vi "name.vi"(0 "Name in":string, 5 "IN VARIANT in":variant) -> (4 "Name":string, 6 "IN VARIANT out":variant)   [LabVIEW 2015]
uses:
  <vilib>/Utility/Data Type/NI_Data Type.lvlib
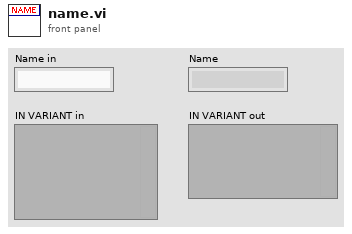
[diagram p1: front panel]
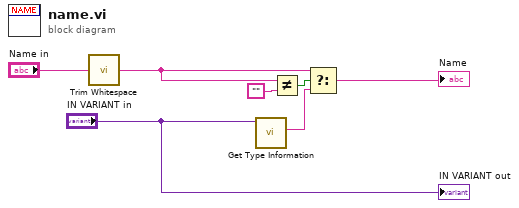
[diagram p0: block diagram]
diagram:
  n1 = call <vilib>:"Trim Whitespace.vi"("string"="Name in") -> ("trimmed string"=w6:string)  [unwired: 1 in]
  n2 = call <vilib>:"Get Type Information.vi"("Variant"="IN VARIANT in") -> ("Name"=w4:string)  [unwired: 6 in, 4 out]
  n3 = Not Equal?(x=w6, y="") -> (x != y?=w2:bool)
  n4 = Select(t=w6, s=w2, f=w4) -> (s? t:f=→"Name":string)
  "IN VARIANT out" <- "IN VARIANT in"
